vi "Read Edit Time Configuration.vi"(8 "error in (no error)":errorcluster, 11 "Session in":refnum<class "Plugin Session.lvclass">) -> (0 "error out":errorcluster, 2 "Edit Time Configuration":string, 3 "Session out":refnum<class "Plugin Session.lvclass">)   [LabVIEW 2021, in "InstrumentStudio Plugin SDK.lvlib" / "Plugin Session.lvclass"]
doc: "Call this VI to read the edit-time configuration string for your plugin panel."
uses:
  Plugin Session.lvclass
  Plugin Session.lvclass/Plugin Session.ctl
  Read Session Id.vi
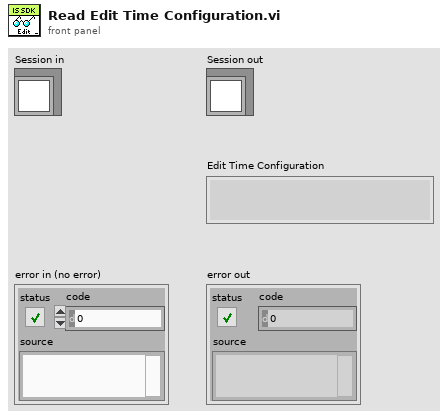
[diagram p1: front panel]
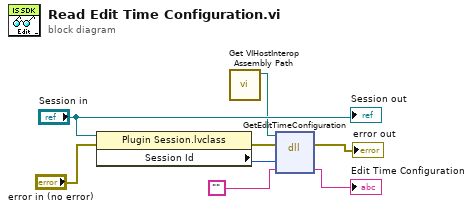
[diagram p0: block diagram]
diagram:
  n1 = property class="Plugin Session.lvclass"(reference="Session in", error in="error in (no error)") -> (error out=w3:errorcluster, "Session Id"=w7:u64)  [unwired: 1 out]
  n2 = call "Get VIHostInterop Assembly Path.vi"() -> ("VIHost.Interop Assembly"=w1:path)  [unwired: 11 in]
  n3 = dll-call lib="C:/ASW/Source/InstrumentStudio/IFDistribution/VIHostPanel/objects/export/targets/win64U/x64/msvc-14.0/debug/NationalInstruments.VIHost.Interop.dll" fn="GetEditTimeConfiguration"(path in=w1, error in=w3, "hostId"=w7, "configuration"="") -> (error out=→"error out":errorcluster, "configuration"=→"Edit Time Configuration":string)  [unwired: 3 in, 1 out]
  "Session out" <- "Session in"
